vi "Exercise1.26-Producer-Consumer-Events.vi"() -> ()   [LabVIEW 2013]
doc: "Use this template to build a producer/consumer design pattern with events to produce queue items. Use this design pattern instead of the User Interface Event Handler pattern for user interfaces when you want to execute code asynchronously in response to an event without slowing the user interface responsiveness."
panel:
  out "Waveform Chart":dbl(graph)
  in  "stop":bool
  in  "OK Button":bool
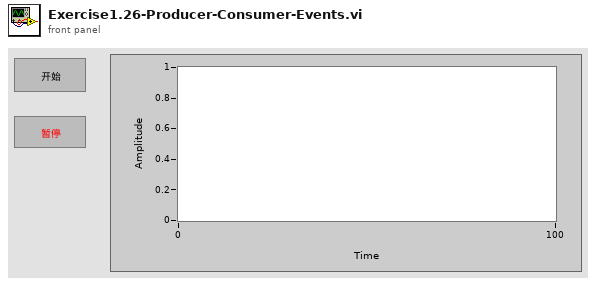
[diagram p1: front panel]
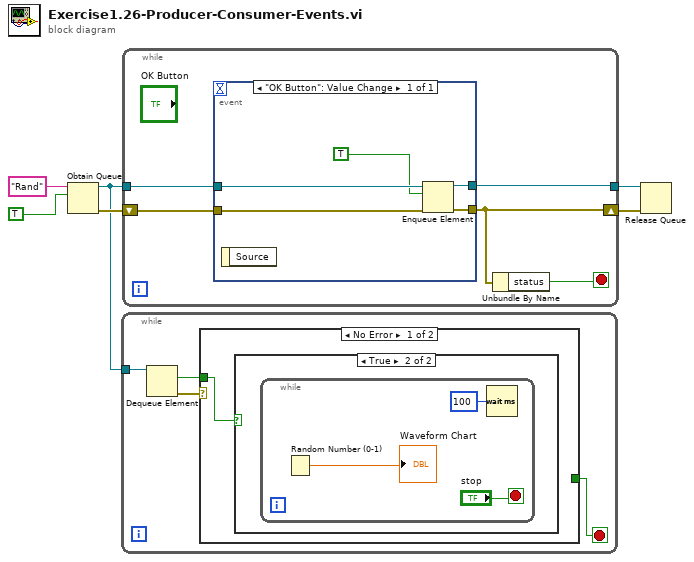
[diagram p0: block diagram]
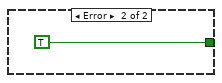
[diagram p3: hidden frame]
diagram:
  n1 = Obtain Queue(name (unnamed)="Rand", element data type=TRUE) -> (queue out=w4:refnum<queue>, error out=w6:errorcluster)  [unwired: 3 in, 1 out]
  n2 = while {
    tunnel: w4 -> [w10]
    stop <- w7 stop-if-true
    n3 = Dequeue Element(queue=w10) -> (element=w8:bool, error out=w9:errorcluster)  [unwired: 2 in, 2 out]
    n4 = case shown="No Error" w9 {
      tunnel: w8 -> [w11 _]
      tunnel: [_ TRUE] -> w7
      frame No Error {
        n5 = case shown="True" w11 {
          frame False {
          }
          frame True {
            n6 = while {
              stop <- "stop" stop-if-true
              n7 = Random Number (0-1)() -> (number: 0 to 1=→"Waveform Chart":dbl)
              n8 = Wait (ms)(milliseconds to wait=u32 100) -> ()  [unwired: 1 out]
            }
          }
        }
      }
      frame Error {
      }
    }
  }
  n9 = while {
    shift-right: [w18] -> w5
    shift-left: w6 -> [w19]
    tunnel: w4 -> [w20]
    tunnel: [w17] -> w1
    stop <- w16 stop-if-true
    n10 = event shown="[0] \"OK Button\": Value Change" {
      selector: _ -> [_]
      dyn-events: _ -> [_]
      timeout: _ -> [_]
      tunnel: w20 -> [w25]
      tunnel: w19 -> [w24]
      tunnel: [w23] -> w18
      tunnel: [w21] -> w17
      event "OK Button": Value Change {
        n11 = event-data() -> ()  [unwired: 1 in, 1 out]
        n12 = Enqueue Element(queue=w25, element=TRUE, error in (no error)=w24) -> (queue out=w21:refnum<queue>, error out=w23:errorcluster)  [unwired: 1 in, 1 out]
      }
    }
    n13 = Unbundle By Name(w18) -> ("status"=w16:bool)
  }
  n14 = Release Queue(queue=w1, error in (no error)=w5) -> ()  [unwired: 1 in, 3 out]
